vi "串口自动测试.vi"(9 "RS485选择":bool, 11 "RS232选择":bool) -> ()   [LabVIEW 2010]
uses:
  <vilib>/Instr/_visa.llb/VISA Configure Serial Port (Instr).vi
  全局量/试验配置信息.vi
  全局量/自动测试结果.vi
  全局量/全局_配置.vi
panel:
  in  "第2路RS485":string
  in  "第1路RS485":string
  in  "第2路RS232":string
  in  "第1路RS232":string
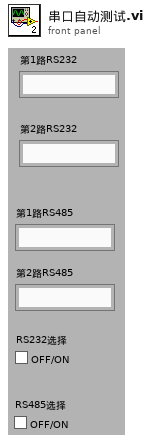
[diagram p1: front panel]
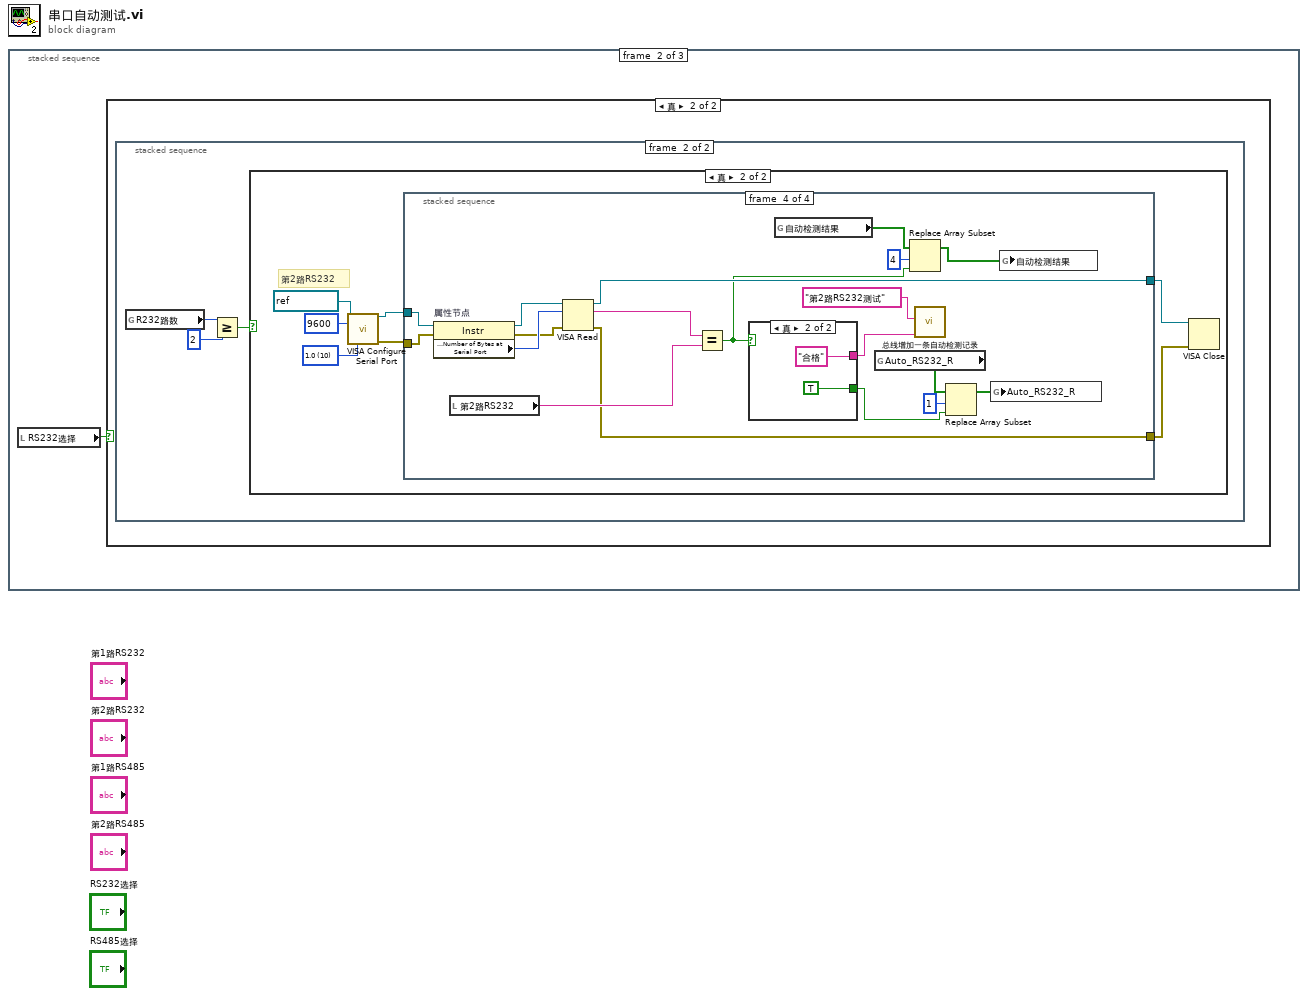
[diagram p0: block diagram]
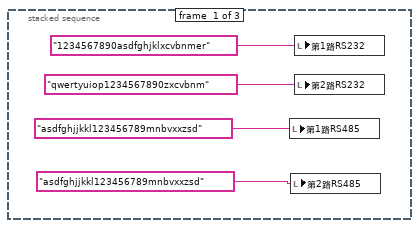
[diagram p2: hidden frame]
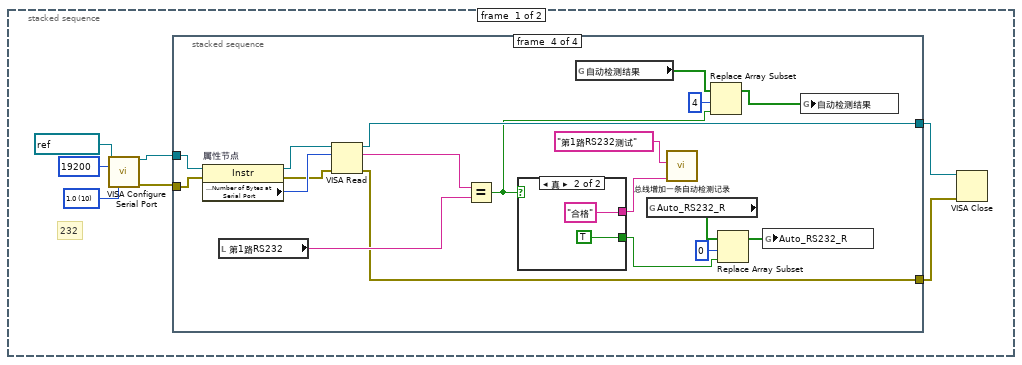
[diagram p4: hidden frame]
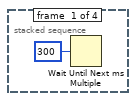
[diagram p5: hidden frame]
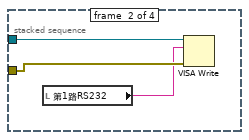
[diagram p6: hidden frame]
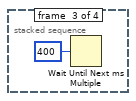
[diagram p7: hidden frame]
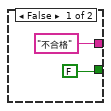
[diagram p8: hidden frame]
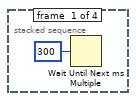
[diagram p10: hidden frame]
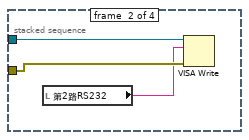
[diagram p11: hidden frame]
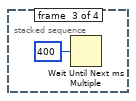
[diagram p12: hidden frame]
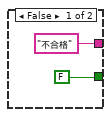
[diagram p13: hidden frame]
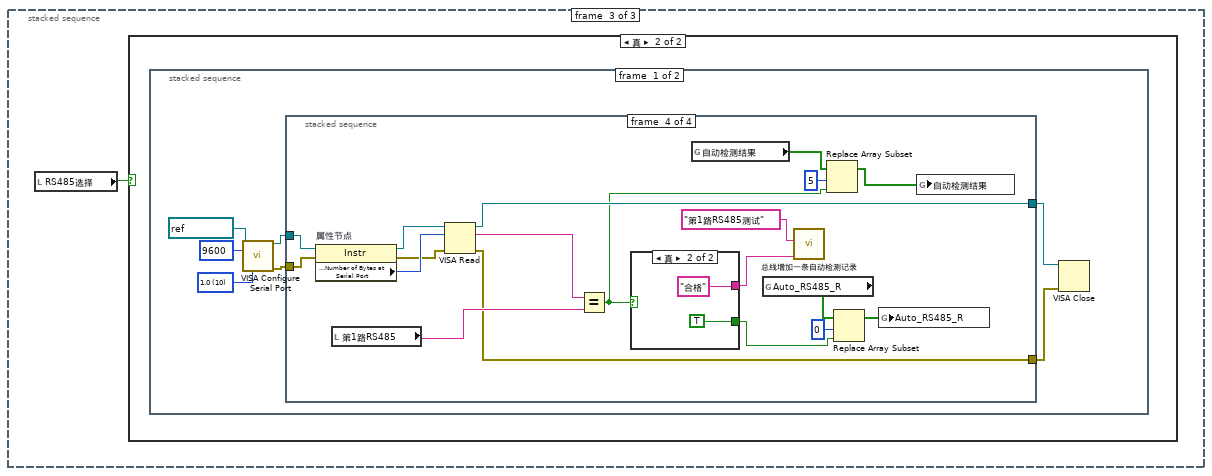
[diagram p14: hidden frame]
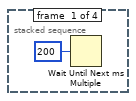
[diagram p16: hidden frame]
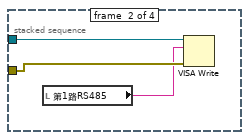
[diagram p17: hidden frame]
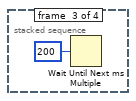
[diagram p18: hidden frame]
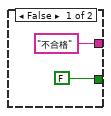
[diagram p19: hidden frame]
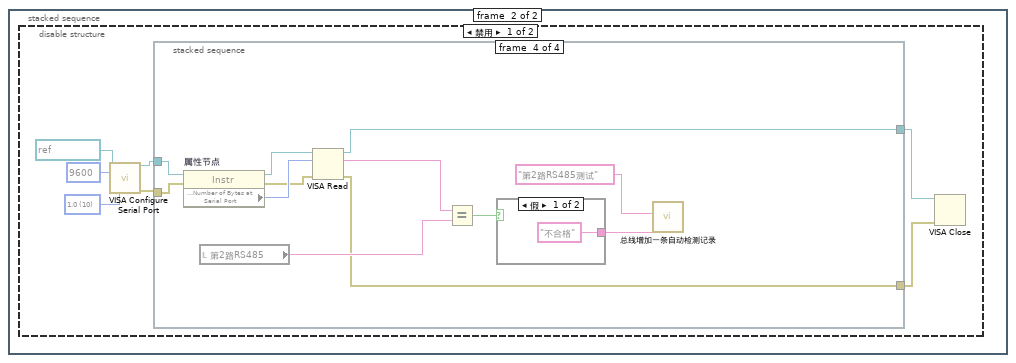
[diagram p20: hidden frame]
diagram:
  n1 = stacked-sequence {
    frame #0 {
      n2 = local write "第1路RS485"("asdfghjjkkl123456789mnbvxxzsd" ("发送字符串_3")) -> ()
      n3 = local write "第2路RS485"("asdfghjjkkl123456789mnbvxxzsd" ("发送字符串_3")) -> ()
      n4 = local write "第1路RS232"("1234567890asdfghjklxcvbnmer" ("发送字符串_1")) -> ()
      n5 = local write "第2路RS232"("qwertyuiop1234567890zxcvbnm" ("发送字符串_2")) -> ()
    }
    frame #1 {
      n6 = local read "RS232选择"() -> (w5:bool)
      n7 = case shown="真" w5 {
        frame False {
        }
        frame True {
          n8 = stacked-sequence {
            frame #0 {
              w8 = u16 10 items=["1.0"=10, "1.5"=15, "2.0"=20] ("stop bits (10: 1 bit)")
              # "232"
              n9 = call-poly "VISA Configure Serial Port"("VISA resource name"=refnum<visa-resource-name> "COM1", "baud rate (9600)"=u32 19200, "stop bits (10: 1 bit)"=w8) -> ("VISA resource name out"=w7:refnum<visa-resource-name>, "error out"=w6:errorcluster)  [unwired: 11 in]
              n10 = stacked-sequence {
                tunnel: w7 -> [_ w16 _ w30]
                tunnel: w6 -> [_ w15 _ w29]
                tunnel: [_ _ _ w32] -> w12
                tunnel: [_ _ _ w31] -> w11
                frame #0 {
                  n11 = Wait Until Next ms Multiple(millisecond multiple=u32 300 ("毫秒倍数")) -> ()  [unwired: 1 out]
                }
                frame #1 {
                  n12 = local read "第1路RS232"() -> (w14:string)
                  n13 = VISA Write(VISA resource name=w16, write buffer=w14, error in (no error)=w15) -> ()  [unwired: 3 out]
                }
                frame #2 {
                  n14 = Wait Until Next ms Multiple(millisecond multiple=u32 400 ("毫秒倍数")) -> ()  [unwired: 1 out]
                }
                frame #3 {
                  n15 = property on="属性节点" class="Instr"(reference=w30, error in=w29) -> (reference out=w36:refnum<visa-resource-name>, error out=w34:errorcluster, "Serial Settings:Number of Bytes at Serial Port"=w35:u32)
                  n16 = local read "第1路RS232"() -> (w33:string)
                  n17 = VISA Read(VISA resource name=w36, byte count=w35, error in (no error)=w34) -> (VISA resource name out=w32:refnum<visa-resource-name>, read buffer=w28:string, error out=w31:errorcluster)  [unwired: 1 out]
                  n18 = Equal?(x=w28, y=w33) -> (x = y?=w18:bool)
                  n19 = case shown="真" w18 {
                    tunnel: ["不合格" "合格"] -> w26
                    tunnel: [FALSE TRUE] -> w22
                    frame False {
                    }
                    frame True {
                    }
                  }
                  n20 = global read "试验配置信息.vi" "自动检测结果"() -> (w19:bool[])
                  n21 = global read "自动测试结果.vi" "Auto_RS232_R"() -> (w25:bool[])
                  n22 = call "总线增加一条自动检测记录.vi"("测试结果"=w26, "测试内容"="第1路RS232测试") -> ()  [unwired: 10 in]
                  n23 = Replace Array Subset(array=w19, new element=w18, index=4 ("索引")) -> (w20:bool[])
                  n24 = Replace Array Subset(array=w25, new element=w22, index=0 ("索引")) -> (w24:bool[])
                  n25 = global write "自动测试结果.vi" "Auto_RS232_R"(w24) -> ()
                  n26 = global write "试验配置信息.vi" "自动检测结果"(w20) -> ()
                }
              }
              n27 = VISA Close(VISA resource name=w12, error in (no error)=w11) -> ()  [unwired: 1 out]
            }
            frame #1 {
              n28 = global read "全局_配置.vi" "R232路数"() -> (w42:u32)
              n29 = Greater Or Equal?(x=w42, y=u32 2) -> (x >= y?=w41:bool)
              n30 = case shown="真" w41 {
                frame False {
                }
                frame True {
                  w46 = u16 10 items=["1.0"=10, "1.5"=15, "2.0"=20] ("stop bits (10: 1 bit)")
                  # "第2路RS232"
                  n31 = call-poly "VISA Configure Serial Port"("VISA resource name"=refnum<visa-resource-name> "COM3", "baud rate (9600)"=u32 9600, "stop bits (10: 1 bit)"=w46) -> ("VISA resource name out"=w49:refnum<visa-resource-name>, "error out"=w50:errorcluster)  [unwired: 11 in]
                  n32 = stacked-sequence {
                    tunnel: w49 -> [_ w54 _ w68]
                    tunnel: w50 -> [_ w53 _ w67]
                    tunnel: [_ _ _ w70] -> w44
                    tunnel: [_ _ _ w69] -> w45
                    frame #0 {
                      n33 = Wait Until Next ms Multiple(millisecond multiple=u32 300 ("毫秒倍数")) -> ()  [unwired: 1 out]
                    }
                    frame #1 {
                      n34 = local read "第2路RS232"() -> (w52:string)
                      n35 = VISA Write(VISA resource name=w54, write buffer=w52, error in (no error)=w53) -> ()  [unwired: 3 out]
                    }
                    frame #2 {
                      n36 = Wait Until Next ms Multiple(millisecond multiple=u32 400 ("毫秒倍数")) -> ()  [unwired: 1 out]
                    }
                    frame #3 {
                      n37 = property on="属性节点" class="Instr"(reference=w68, error in=w67) -> (reference out=w74:refnum<visa-resource-name>, error out=w72:errorcluster, "Serial Settings:Number of Bytes at Serial Port"=w73:u32)
                      n38 = local read "第2路RS232"() -> (w71:string)
                      n39 = VISA Read(VISA resource name=w74, byte count=w73, error in (no error)=w72) -> (VISA resource name out=w70:refnum<visa-resource-name>, read buffer=w64:string, error out=w69:errorcluster)  [unwired: 1 out]
                      n40 = Equal?(x=w64, y=w71) -> (x = y?=w56:bool)
                      n41 = case shown="真" w56 {
                        tunnel: ["不合格" "合格"] -> w65
                        tunnel: [FALSE TRUE] -> w60
                        frame False {
                        }
                        frame True {
                        }
                      }
                      n42 = global read "试验配置信息.vi" "自动检测结果"() -> (w57:bool[])
                      n43 = global read "自动测试结果.vi" "Auto_RS232_R"() -> (w63:bool[])
                      n44 = Replace Array Subset(array=w57, new element=w56, index=4 ("索引")) -> (w58:bool[])
                      n45 = call "总线增加一条自动检测记录.vi"("测试结果"=w65, "测试内容"="第2路RS232测试") -> ()  [unwired: 10 in]
                      n46 = Replace Array Subset(array=w63, new element=w60, index=1 ("索引")) -> (w62:bool[])
                      n47 = global write "自动测试结果.vi" "Auto_RS232_R"(w62) -> ()
                      n48 = global write "试验配置信息.vi" "自动检测结果"(w58) -> ()
                    }
                  }
                  n49 = VISA Close(VISA resource name=w44, error in (no error)=w45) -> ()  [unwired: 1 out]
                }
              }
            }
          }
        }
      }
    }
    frame #2 {
      n50 = local read "RS485选择"() -> (w79:bool)
      n51 = case shown="真" w79 {
        frame False {
        }
        frame True {
          n52 = stacked-sequence {
            frame #0 {
              w84 = u16 10 items=["1.0"=10, "1.5"=15, "2.0"=20] ("stop bits (10: 1 bit)")
              n53 = call-poly "VISA Configure Serial Port"("VISA resource name"=refnum<visa-resource-name> "COM4", "baud rate (9600)"=u32 9600, "stop bits (10: 1 bit)"=w84) -> ("VISA resource name out"=w81:refnum<visa-resource-name>, "error out"=w80:errorcluster)  [unwired: 11 in]
              n54 = stacked-sequence {
                tunnel: w81 -> [_ w90 _ w104]
                tunnel: w80 -> [_ w89 _ w103]
                tunnel: [_ _ _ w106] -> w86
                tunnel: [_ _ _ w105] -> w85
                frame #0 {
                  n55 = Wait Until Next ms Multiple(millisecond multiple=u32 200 ("毫秒倍数")) -> ()  [unwired: 1 out]
                }
                frame #1 {
                  n56 = local read "第1路RS485"() -> (w88:string)
                  n57 = VISA Write(VISA resource name=w90, write buffer=w88, error in (no error)=w89) -> ()  [unwired: 3 out]
                }
                frame #2 {
                  n58 = Wait Until Next ms Multiple(millisecond multiple=u32 200 ("毫秒倍数")) -> ()  [unwired: 1 out]
                }
                frame #3 {
                  n59 = property on="属性节点" class="Instr"(reference=w104, error in=w103) -> (reference out=w110:refnum<visa-resource-name>, error out=w108:errorcluster, "Serial Settings:Number of Bytes at Serial Port"=w109:u32)
                  n60 = local read "第1路RS485"() -> (w107:string)
                  n61 = VISA Read(VISA resource name=w110, byte count=w109, error in (no error)=w108) -> (VISA resource name out=w106:refnum<visa-resource-name>, read buffer=w102:string, error out=w105:errorcluster)  [unwired: 1 out]
                  n62 = Equal?(x=w102, y=w107) -> (x = y?=w92:bool)
                  n63 = case shown="真" w92 {
                    tunnel: ["不合格" "合格"] -> w100
                    tunnel: [FALSE TRUE] -> w96
                    frame False {
                    }
                    frame True {
                    }
                  }
                  n64 = global read "试验配置信息.vi" "自动检测结果"() -> (w93:bool[])
                  n65 = global read "自动测试结果.vi" "Auto_RS485_R"() -> (w99:bool[])
                  n66 = call "总线增加一条自动检测记录.vi"("测试结果"=w100, "测试内容"="第1路RS485测试") -> ()  [unwired: 10 in]
                  n67 = Replace Array Subset(array=w93, new element=w92, index=5 ("索引")) -> (w94:bool[])
                  n68 = Replace Array Subset(array=w99, new element=w96, index=0 ("索引")) -> (w98:bool[])
                  n69 = global write "自动测试结果.vi" "Auto_RS485_R"(w98) -> ()
                  n70 = global write "试验配置信息.vi" "自动检测结果"(w94) -> ()
                }
              }
              n71 = VISA Close(VISA resource name=w86, error in (no error)=w85) -> ()  [unwired: 1 out]
            }
            frame #1 {
              n72 = disable-structure shown="禁用" {
                frame Disabled {
                  w121 = u16 10 items=["1.0"=10, "1.5"=15, "2.0"=20] ("stop bits (10: 1 bit)")
                  n73 = call-poly "VISA Configure Serial Port"("VISA resource name"=refnum<visa-resource-name> "COM5", "baud rate (9600)"=u32 9600, "stop bits (10: 1 bit)"=w121) -> ("VISA resource name out"=w116:refnum<visa-resource-name>, "error out"=w115:errorcluster)  [unwired: 11 in]
                  n74 = stacked-sequence {
                    tunnel: w116 -> [_ w125 _ w131]
                    tunnel: w115 -> [_ w124 _ w130]
                    tunnel: [_ _ _ w133] -> w118
                    tunnel: [_ _ _ w132] -> w117
                    frame #0 {
                      n75 = Wait Until Next ms Multiple(millisecond multiple=u32 200 ("毫秒倍数")) -> ()  [unwired: 1 out]
                    }
                    frame #1 {
                      n76 = local read "第2路RS485"() -> (w123:string)
                      n77 = VISA Write(VISA resource name=w125, write buffer=w123, error in (no error)=w124) -> ()  [unwired: 3 out]
                    }
                    frame #2 {
                      n78 = Wait Until Next ms Multiple(millisecond multiple=u32 200 ("毫秒倍数")) -> ()  [unwired: 1 out]
                    }
                    frame #3 {
                      n79 = property on="属性节点" class="Instr"(reference=w131, error in=w130) -> (reference out=w137:refnum<visa-resource-name>, error out=w135:errorcluster, "Serial Settings:Number of Bytes at Serial Port"=w136:u32)
                      n80 = local read "第2路RS485"() -> (w134:string)
                      n81 = VISA Read(VISA resource name=w137, byte count=w136, error in (no error)=w135) -> (VISA resource name out=w133:refnum<visa-resource-name>, read buffer=w129:string, error out=w132:errorcluster)  [unwired: 1 out]
                      n82 = Equal?(x=w129, y=w134) -> (x = y?=w138:bool)
                      n83 = case shown="假" w138 {
                        tunnel: ["不合格" "合格"] -> w127
                        frame False {
                        }
                        frame True {
                        }
                      }
                      n84 = call "总线增加一条自动检测记录.vi"("测试结果"=w127, "测试内容"="第2路RS485测试") -> ()  [unwired: 10 in]
                    }
                  }
                  n85 = VISA Close(VISA resource name=w118, error in (no error)=w117) -> ()  [unwired: 1 out]
                }
                frame Enabled {
                }
              }
            }
          }
        }
      }
    }
  }
